vi "ENVIOS DE NOME-SERVER.vi"() -> ()   [LabVIEW 2019]
panel:
  in  "stop":bool
  in  "NOMES":string[](array[string])
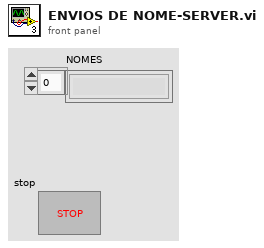
[diagram p1: front panel]
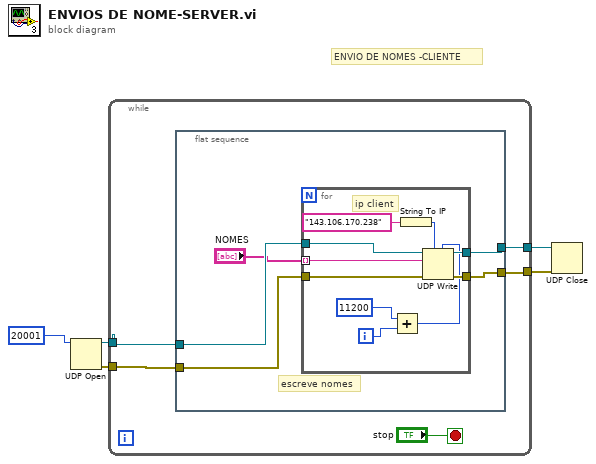
[diagram p0: block diagram]
diagram:
  # "ENVIO DE NOMES -CLIENTE"
  n1 = UDP Open(11:u16 20001 ("port")) -> (port=w2:refnum<k16>, 0:w3:errorcluster)  [unwired: 4 in, 1 out]
  n2 = while {
    tunnel: [w9] -> w5
    tunnel: [w8] -> w4
    tunnel: w3 -> [w7]
    tunnel: w2 -> [w6]
    stop <- "stop" stop-if-true
    n3 = flat-sequence {
      tunnel: [w15] -> w9
      tunnel: [w14] -> w8
      tunnel: w7 -> [w13]
      tunnel: w6 -> [w12]
      frame #0 {
        # "escreve nomes"
        n4 = for {
          tunnel: "NOMES" -> [w21] mode=indexing
          tunnel: [w25] -> w14
          tunnel: [w24] -> w15
          tunnel: w13 -> [w17]
          tunnel: w12 -> [w16]
          i -> [w20]
          # "ip client"
          n5 = Add(x=u16 11200 ("port or service name"), y=w20) -> (x+y=w18:i32)
          n6 = String To IP(1:"143.106.170.238" ("name")) -> (0:w23:u32)
          n7 = UDP Write(address=w23, port or service name=w18, connection ID=w16, data in=w21, 8:w17) -> (error out=w24:errorcluster, 3:w25:refnum<k16>)  [unwired: 1 in]
        }
      }
    }
  }
  n8 = UDP Close(connection ID=w4, 8:w5) -> ()  [unwired: 2 out]
